vi "Write SettlingTime.vi"(8 "error in (no error)":errorcluster, 10 "SettlingTime":dbl, 11 "PmuTestFunctions in":refnum<class "PmuTestFunctions.lvclass">) -> (0 "error out":errorcluster, 3 "PmuTestFunctions out":refnum<class "PmuTestFunctions.lvclass">)   [LabVIEW 2018, in "Functions.lvlib" / "PmuTestFunctions.lvclass"]
uses:
  PmuTestFunctions.lvclass
  PmuTestFunctions.lvclass/PmuTestFunctions.ctl
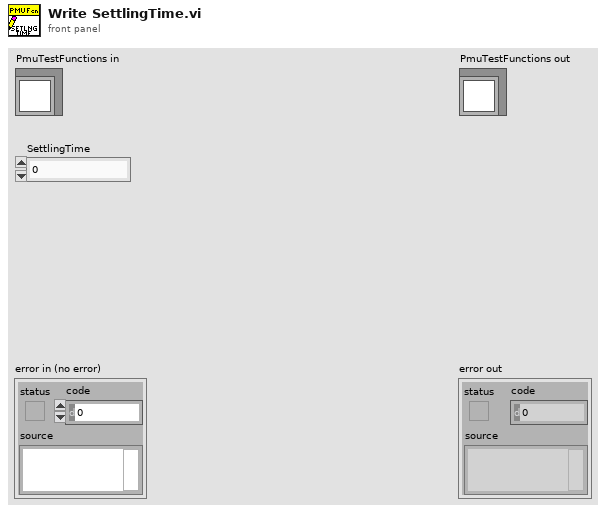
[diagram p1: front panel]
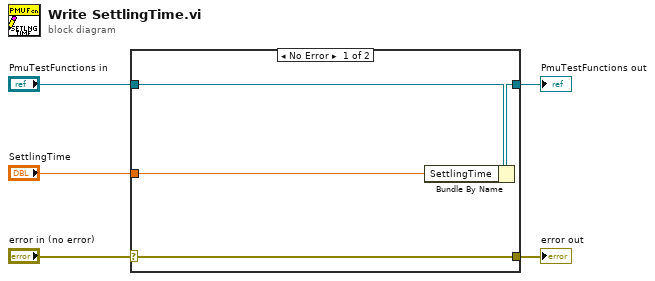
[diagram p0: block diagram]
diagram:
  n1 = case shown="No Error" "error in (no error)" {
    selector: "error in (no error)" -> [w9 w10]
    tunnel: [w9 w10] -> w4
    tunnel: [w7 w11] -> w2
    tunnel: "PmuTestFunctions in" -> [w8 w11]
    tunnel: "SettlingTime" -> [w6 _]
    frame No Error {
      n2 = Bundle By Name(cluster=w8, "SettlingTime"=w6) -> (w7:refnum<class "PmuTestFunctions.lvclass">)
    }
    frame Error {
    }
  }
  "error out" <- w4
  "PmuTestFunctions out" <- w2
